vi "radius_turn.vi"() -> ()   [LabVIEW 2017]
panel:
  in  "Radius":dbl(slide)=801.2422360248447 scale=0.0..1000.0
  in  "Stop Button":bool
  in  "Spedd":dbl(slide)=0.009006211180124225 scale=0.0..0.1
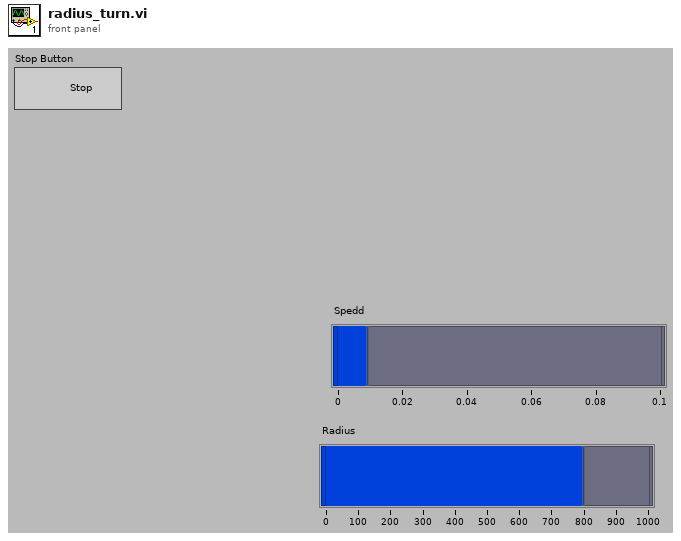
[diagram p1: front panel]
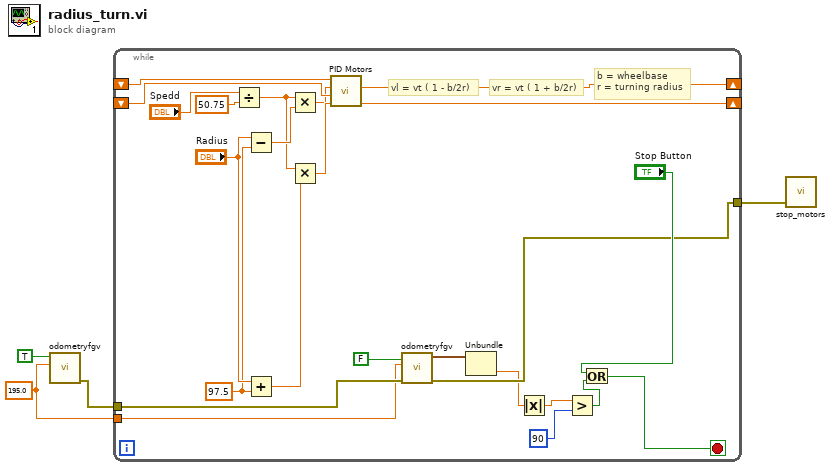
[diagram p0: block diagram]
diagram:
  w1 = 195.0 ("wheelbase")
  n1 = call "odometryfgv.vi"("wheelbase"=w1, "Reset"=TRUE) -> ("error out"=w2:errorcluster)  [unwired: 6 in, 2 out]
  n2 = while {
    shift-right: [w28] -> _
    shift-left: _ -> [w27]
    shift-right: [w26] -> _
    shift-left: _ -> [w25]
    tunnel: [w12] -> w4
    tunnel: w2 -> [w13]
    tunnel: w1 -> [w10]
    stop <- w14 stop-if-true
    w21 = 97.5
    # "b = wheelbase\nr = turning radius"
    # "vr = vt ( 1 + b/2r)"
    # "vl = vt ( 1 - b/2r)"
    n3 = Divide(x="Spedd", y=50.75) -> (x/y=w18:dbl)
    n4 = Subtract(x="Radius", y=w21) -> (x-y=w19:dbl)
    n5 = Add(x="Radius", y=w21) -> (x+y=w20:dbl)
    n6 = Multiply(x=w18, y=w19) -> (x*y=w16:dbl)
    n7 = Multiply(x=w18, y=w20) -> (x*y=w17:dbl)
    n8 = call "PID Motors.vi"("input B"=w17, "Speed B"=w25, "input A"=w16, "Speed A"=w27) -> ("output B"=w26:dbl, "output A"=w28:dbl)  [unwired: 2 out]
    n9 = call "odometryfgv.vi"("error in (no error)"=w13, "wheelbase"=w10, "Reset"=FALSE) -> ("error out"=w12:errorcluster, "X, Y, BEARING"=w9:cluster{dbl, dbl, dbl})  [unwired: 5 in, 1 out]
    n10 = Unbundle(w9) -> (w8:dbl)  [unwired: 2 out]
    n11 = Absolute Value(x=w8) -> (abs(x)=w6:dbl)
    n12 = Greater?(x=w6, y=90) -> (0:w7:bool)
    n13 = Or(x="Stop Button", y=w7) -> (x .or. y?=w14:bool)
  }
  n14 = call "stop_motors.vi"("error in (no error)"=w4) -> ()  [unwired: 4 in, 1 out]
